vi "Dashboard Main.vi"() -> ()   [LabVIEW 2013]
uses:
  Robot Code/2014 Initial Robot/Shooter State Enum.ctl
  <vilib>/event_ctls.llb/eventvkey.ctl
  <vilib>/Rock Robotics/WPI/Dashboard/WPI_DashboardLogging Global.vi
  <vilib>/Utility/config.llb/Write Key (String).vi
  <vilib>/Utility/config.llb/Write Key (I32).vi
  <vilib>/Utility/config.llb/NI_LVConfig.lvlib
panel:
  out "Image Message":string="Timeout in Camera Communications"
  in  "Rec Mode":enum32{"Stop", "Record", "Playback"}(radio)
  in  "Dashboard Tab":T1(tab)
  in  "Camera Settings":T2={"Frame Rate"=30, "Compression"=30, "Size"=1} {"Frame Rate" scale=1.0..30.0; "Size" items=["640x480", "320x240", "160x120"]}
  out "MotorSliders R":cluster{"MotorSlide1":dbl, "MotorSlide2":dbl} {"MotorSlide2" scale=-1.0..1.0 scale format="%#_2e"; "MotorSlide1" scale=-1.0..1.0 scale format="%#_2e"}
  out "MotorChart R":cluster{"Numeric":dbl, "Numeric":dbl}(graph)
  out "MotorSliders L":T3 {"MotorSlide4 2" scale=0.0..14.0 scale format="%#_2e"; "MotorSlide2" scale=-1.0..1.0 scale format="%#_2e"; "MotorSlide1" scale=-1.0..1.0 scale format="%#_2e"}
  out "MotorChart L":T4(graph)
  out "JS1 Z":dbl(slide) scale=-1.0..1.0 scale format="%#_2e"
  out "Joystick 1":cluster{"X":dbl, "Y":dbl}[](graph)
  out "JS Buttons 1":T5
  out "JS2 Z":dbl(slide) scale=-1.0..1.0 scale format="%#_2e"
  out "Joystick 2":cluster{"X":dbl, "Y":dbl}[](graph)
  out "JS Buttons 2":T5
  out "Mode":T6(ring)=enum."Auto Disabled"
  out "Camera IP":string
  in  "DB Camera Config":bool
  out "fps":dbl format="%#.1g"
  out "Mbps":dbl format="%#.1g"
  out "Mbps 2":bool
  out "LED 1":bool
  out "Shooter":bool
  in  "ShotDrawSpeed":dbl format="%#_13g"
  in  "Pass Speed":dbl=1.0
  in  "Capture Speed":dbl=-1.0
  out "Pass":bool
  out "Collection Motors\nCapture":bool
  out "Upper":bool
  out "Limit Switches\nLower":bool
  in  "ArmSpeedDown":dbl=0.2
  in  "ArmSpeedUp":dbl=0.35
  out "ArmPosition":string
  out "CurrentPosition":dbl
  in  "TrussPosition":dbl=100.0
  in  "ShootPosition":dbl=61.0
  in  "PickUpPosition":dbl=12.0
  out "YAxisAccel":dbl
  in  "SecToFull":dbl=0.5 min=0.2 max=2.0
  out "ArmMotorValue":dbl
  out "Shooter State":T7
  in  "Checkbox 2":bool
  in  "Checkbox 1":bool
  in  "Test Slider":dbl(slide) scale=0.0..100.0 scale format="%#_3g"
  in  "On/Off":bool caption="Solenoid"
  in  "Test Name":u16(ring) items=["Select the test to run...", "Example Test", "-------------------------------", "List of tests is built in robot code.", "Replace with your own automated tests."]
  in  "Test Tree":string(tree)
  in  "Motor":cluster{"Value":dbl, "Enable":bool} {"Value" scale=-1.0..1.0 scale format="%#_3g"}
  out "Progress":T8 {"Test Progress" scale=0.0..100.0}
  in  "Rev/Fwd":cluster{"Forward":bool, "Reverse":bool}
  in  "Test Ring":u16(ring) items=["Auto", "Fixed indoor", "Fixed outdoor 1", "Fixed outdoor 2", "Fixed fluorescent 1", "Fixed fluorescent 2", "Hold current"]
  out "Potentiometer Value":dbl
  in  "Bottom Arm Value":dbl=1.43
  in  "Listbox":i32(listbox)
  out "Tree":string(tree)
  out "Camera Image":T9(plugin-control)
  in  "Enable":bool
  # "Left"
  # "Front"
  # "Right"
  # "Battery"
  # "This tab is a great place for autonomous settings and validation.\nCustomize by placing controls and indicators here and name to\nmatch Dashboard Variables on robot."
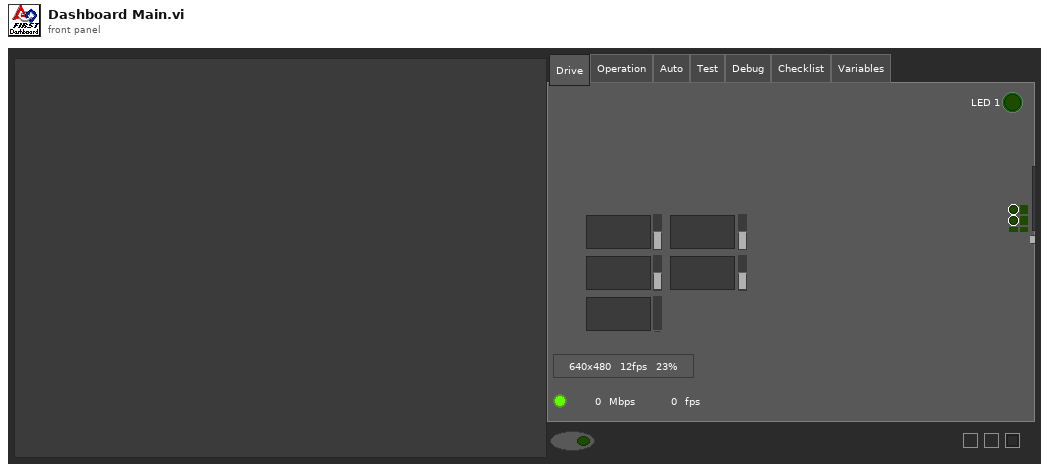
[diagram p1: front panel]
types:
  T1 = enum32{"Drive", "Operation", "Auto", "Test", "Debug", "Checklist", "Variables"}
  T2 = cluster{"Frame Rate":i32, "Compression":i32, "Size":u16}
  T3 = cluster{"MotorSlide1":dbl, "MotorSlide2":dbl, "MotorSlide4 2":dbl}
  T4 = cluster{"Numeric":dbl, "Numeric":dbl, "Battery":sgl}
  T5 = cluster{bool, bool, bool, bool, bool, bool, bool, bool, bool, bool, bool, bool}
  T6 = enum8{"Tele-Op Disabled", "Tele-Op Enabled", "Auto Disabled", "Auto Enabled", "Test Disabled", "Test Enabled", ""}
  T7 = typedef "Shooter State Enum.ctl" = enum16{"Ready", "Fired", "DrawingToReady"}
  T8 = cluster{"Test Progress":u8, "Test Progress Text":string}
  T9 = typedef "IMAQ Image.ctl" = refnum<image>
  T10 = enum32{"Drive", "Operation", "Auto", "Test", "Checklist", "Variables"}
  T11 = typedef "Image Type" = u32
  T12 = cluster{"Digital Inputs":bool[], "Digital Outputs":bool[]}
  T13 = cluster{"Competition mode":bool, "Robot Link":bool, "Autonomous":bool, "Enabled":bool, "E-Stop":bool, "Simulated":bool, "TestMode":bool, "Docked Window":bool}
  T14 = cluster{"Boolean Array[0]":bool, "Boolean Array[1]":bool, "Boolean Array[2]":bool, "Boolean Array[3]":bool, "Boolean Array[4]":bool, "Boolean Array[5]":bool, "Boolean Array[6]":bool, "Boolean Array[7]":bool, "Boolean Array[8]":bool, "Boolean Array[9]":bool, "Boolean Array[10]":bool, "Boolean Array[11]":bool}
  T15 = typedef "NI_LVConfig.lvlib/Config Data RefNum.ctl" = refnum<k1>
  T16 = typedef "eventvkey.ctl" = enum16{"ASCII", "Enter", "Return", "Shift", "Ctrl", "Alt", "Cmd", "Opt", "Caps", "NumLock", "Clear", "Break", "Up", "Down", "Left", "Right", "Insert", "Delete", "Home", "End", "PageUp", "PageDown", "Escape", "Help", "Pause", "ScrollLock", "F1", "F2", "F3", "F4", "F5", "F6", "F7", "F8", "F9", "F10", "F11", "F12", "F13", "F14", "F15", "F16", "F17", "F18", "F19", "F20", "F21", "F22", "F23", "F24", "Play", "VolumeUp", "VolumeDown", "Mute", "Two Byte Char"}
  T17 = cluster{"Image Size":bool, "Image Type":bool, "Pixel Value":bool, "ROI Information":bool, "Zoom Factor":bool}
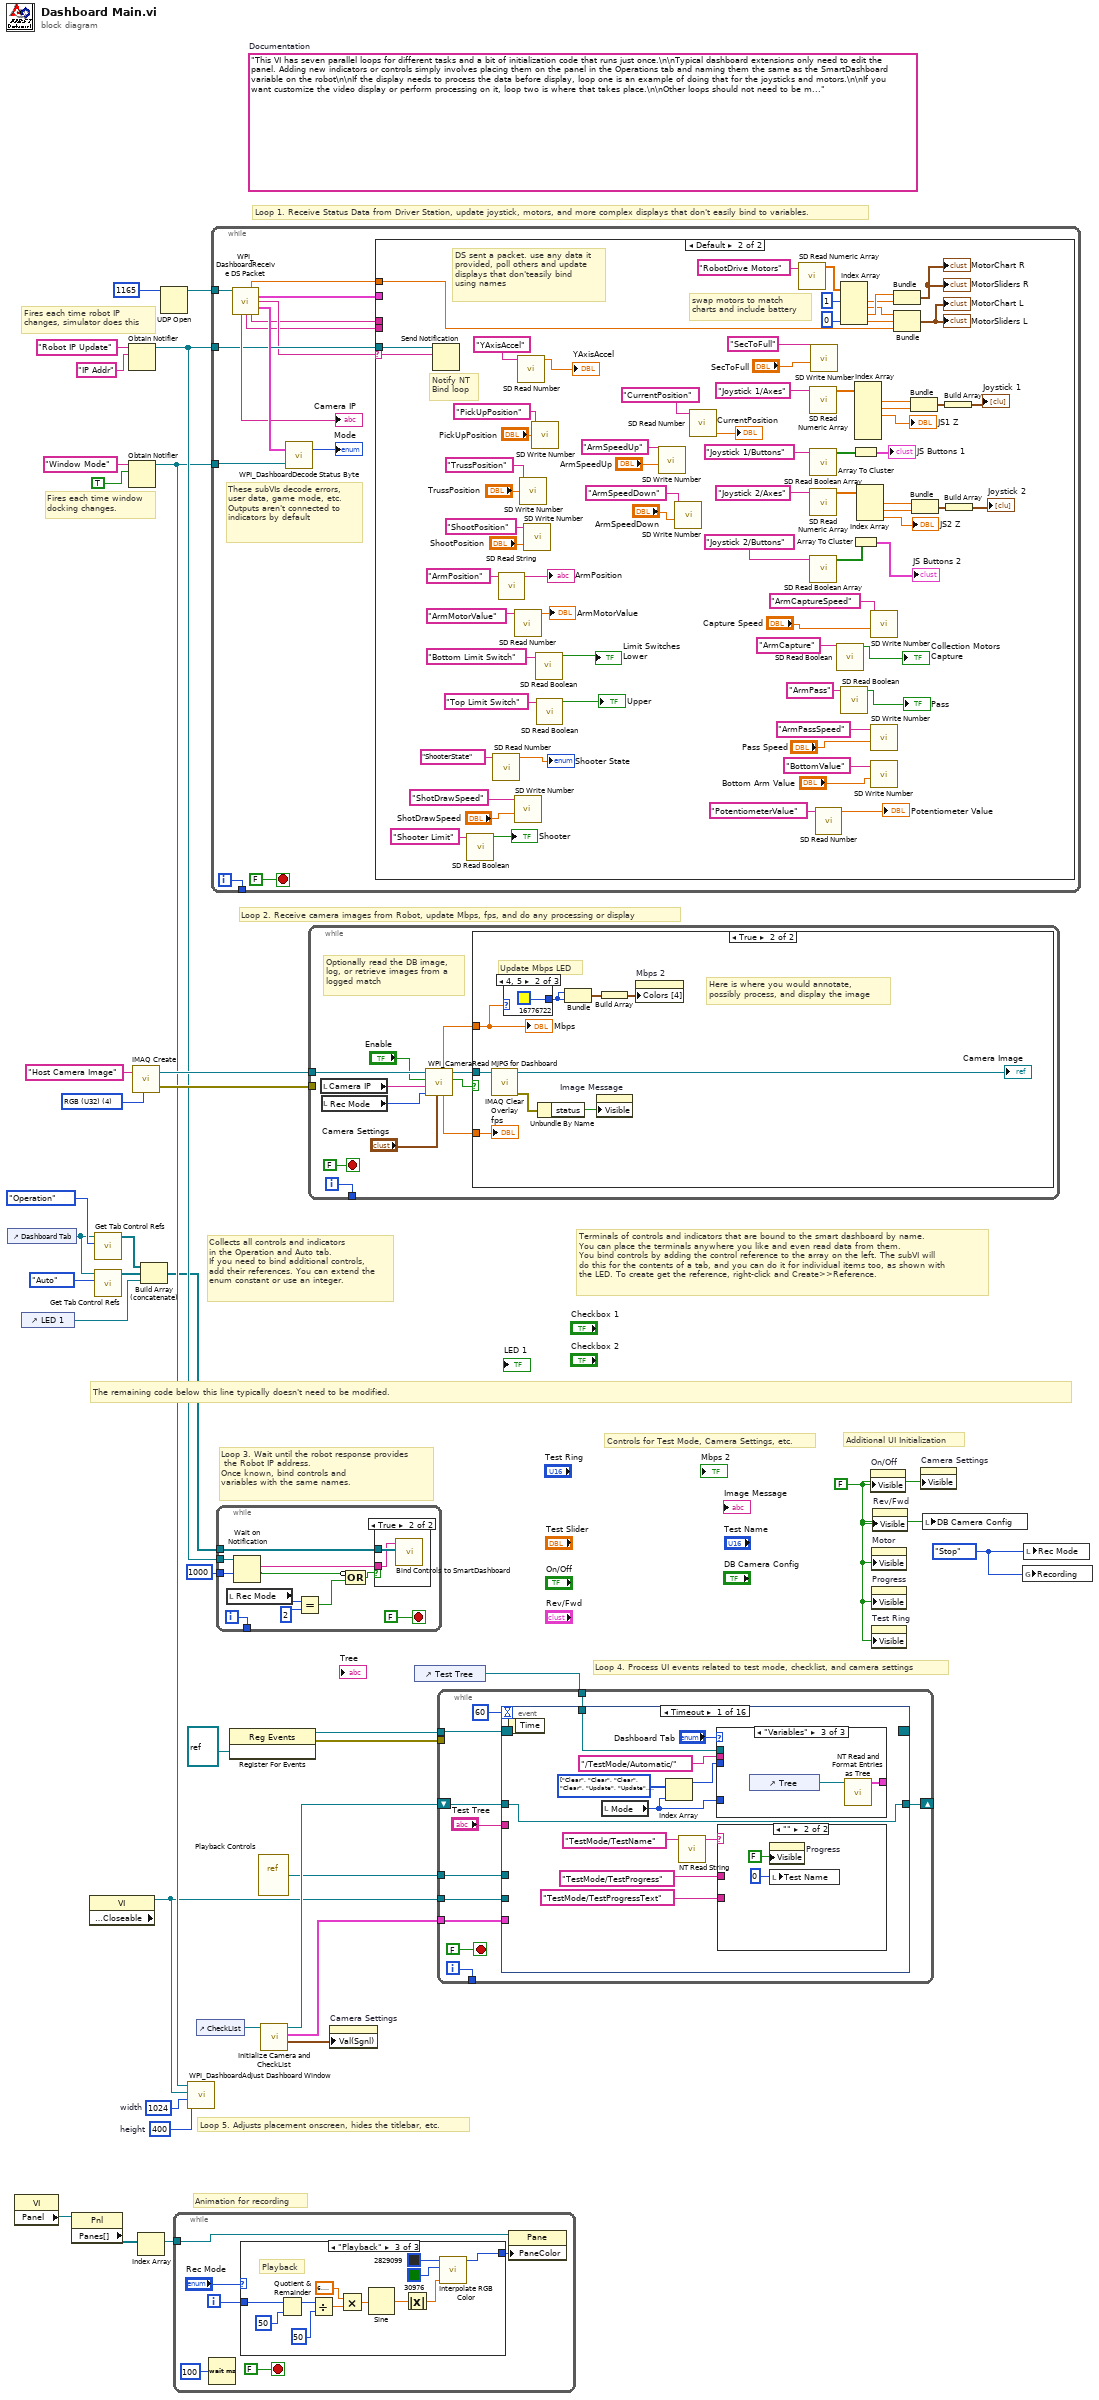
[diagram p0: block diagram]
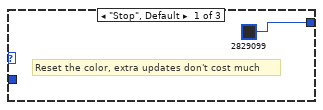
[diagram p2: hidden frame]
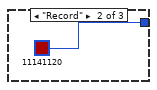
[diagram p3: hidden frame]
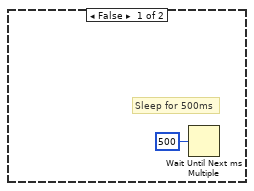
[diagram p5: hidden frame]
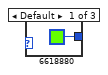
[diagram p6: hidden frame]
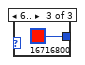
[diagram p7: hidden frame]
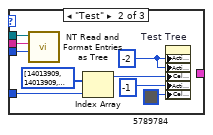
[diagram p9: hidden frame]
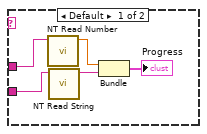
[diagram p10: hidden frame]
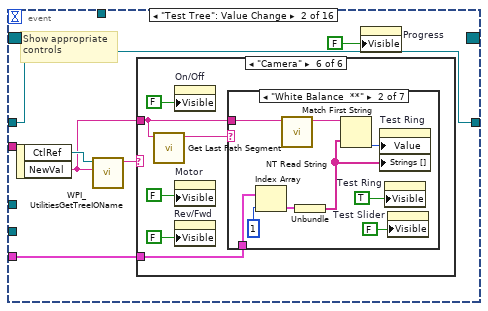
[diagram p11: hidden frame]
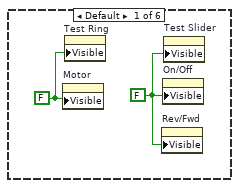
[diagram p12: hidden frame]
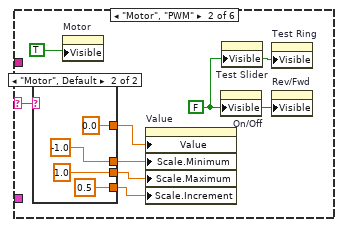
[diagram p13: hidden frame]
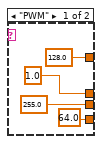
[diagram p14: hidden frame]
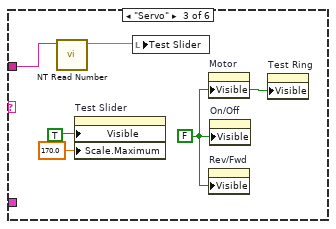
[diagram p15: hidden frame]
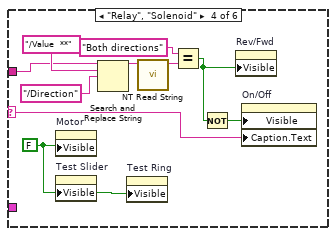
[diagram p16: hidden frame]
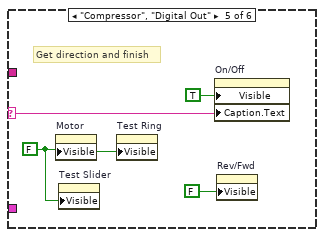
[diagram p17: hidden frame]
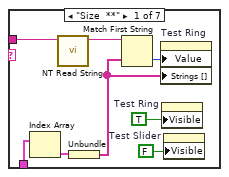
[diagram p18: hidden frame]
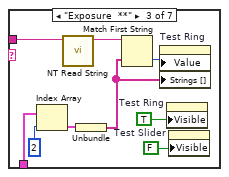
[diagram p19: hidden frame]
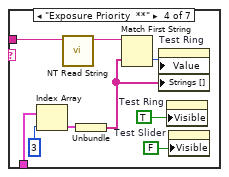
[diagram p20: hidden frame]
diagram:
  w8 = enum32{"Stop", "Record", "Playback"}."Stop" ("Rec Mode")
  w11 = 400  # height
  w12 = 1024  # width
  w25 = FALSE ("Visible")
  (unwired) "This VI has seven parallel loops for different tasks and a bit of initialization code that runs just once.\n\nTypical dashboard extensions only need to edit the panel. Adding new indicators or controls simply involves placing them on the panel in the Operations tab and naming them the same as the SmartDashboard variable on the robot\n\nIf the display needs to process the data before display, loop one is an example of doing that for the joysticks and motors.\n\nIf you want customize the video display or perform processing on it, loop two is where that takes place.\n\nOther loops should not need to be modified. They are pretty standard, and document the task they perform."  # Documentation
  w35 = T11 4 items=["Grayscale (U8)", "Grayscale (I16)", "Grayscale (SGL)", "Complex (CSG)", "RGB (U32)", "HSL (U32)", "RGB (U64)"] ("Image Type")
  # "Controls for Test Mode, Camera Settings, etc."
  # "Additional UI Initialization"
  # "Animation for recording"
  # "Fires each time robot IP\nchanges, simulator does this"
  # "Fires each time window\ndocking changes."
  # "Collects all controls and indicators\nin the Operation and Auto tab.\nIf you need to bind additional controls,\nadd their references. You can extend the\nenum constant or use an integer."
  # "The remaining code below this line typically doesn't need to be modified."
  # "Loop 4. Process UI events related to test mode, checklist, and camera settings"
  # "Terminals of controls and indicators that are bound to the smart dashboard by name.\nYou can place the terminals anywhere you like and even read data from them.\nYou bind controls by adding the control reference to the array on the left. The subVI will\ndo this for the contents of a tab, and you can do it for individual items too, as shown with\nthe LED. To create get the reference, right-click and Create>>Reference."
  # "Loop 3. Wait until the robot response provides\n the Robot IP address.\nOnce known, bind controls and\nvariables with the same names."
  # "Loop 5. Adjusts placement onscreen, hides the titlebar, etc."
  # "Loop 1. Receive Status Data from Driver Station, update joystick, motors, and more complex displays that don't easily bind to variables."
  # "Loop 2. Receive camera images from Robot, update Mbps, fps, and do any processing or display"
  n1 = control-ref of="Dashboard Tab"() -> (w6:refnum<vi>)
  n2 = property class="VI"() -> ("Panel"=w19:refnum<vi>)  [unwired: 2 in, 2 out]
  n3 = control-ref of="LED 1"() -> (w1:refnum<vi>)
  n4 = property class="Pnl"(reference=w19) -> ("Panes[]"=w20:refnum<vi>[])  [unwired: 1 in, 2 out]
  n5 = property class="VI" props=["Front Panel.Closeable"]() -> (reference out=w7:refnum<vi>)  [unwired: 2 in, 2 out]
  n6 = call <vilib>:"Get Tab Control Refs.vi"("Page Index"=T10."Operation" ("Dashboard Tab"), "TabControl in"=w6) -> ("ControlsOnPage"=w4:refnum<vi>[])  [unwired: 9 in]
  n7 = call <vilib>:"Get Tab Control Refs.vi"("Page Index"=T10."Auto" ("Dashboard Tab"), "TabControl in"=w6) -> ("ControlsOnPage"=w5:refnum<vi>[])  [unwired: 9 in]
  n8 = Obtain Notifier(name (unnamed)="Robot IP Update", notification data type="IP Addr" ("name (unnamed)")) -> (notifier out=w29:refnum<notifier>)  [unwired: 2 in, 2 out]
  n9 = Obtain Notifier(name (unnamed)="Window Mode", notification data type=TRUE) -> (notifier out=w10:refnum<notifier>)  [unwired: 2 in, 2 out]
  n10 = call "IMAQ Create"("Image Name"="Host Camera Image", "Image Type"=w35) -> ("New Image"=w33:T9, "error out"=w32:errorcluster)  [unwired: 2 in, 1 out]
  n11 = Index Array(array=w20) -> (element=w18:refnum<vi>)  [unwired: 1 in]
  n12 = Build Array (concatenate)(w4, w5, w1) -> (w3:refnum<vi>[])
  n13 = UDP Open(11:u16 1165 ("port")) -> (port=w36:refnum<k16>)  [unwired: 2 in, 4 out]
  n14 = while {
    tunnel: w18 -> [w39]
    i -> [w42]
    stop <- FALSE stop-if-true
    n15 = Wait (ms)(milliseconds to wait=u32 100) -> ()  [unwired: 1 out]
    n16 = case shown="\"Playback\"" "Rec Mode" {
      tunnel: w42 -> [_ _ w57]
      tunnel: [u32 2829099 ("Base Color") u32 11141120 ("Target Color") w46] -> w38
      frame "Stop", Default {
        # "Reset the color, extra updates don't cost much"
      }
      frame "Record" {
      }
      frame "Playback" {
        # "Playback"
        n17 = Quotient & Remainder(x=w57, y=u32 50 ("milliseconds to wait")) -> (x-y*floor(x/y)=w53:u32)  [unwired: 1 out]
        n18 = Divide(x=w53, y=u32 50 ("milliseconds to wait")) -> (x/y=w50:dbl)
        n19 = Multiply(x=6.283185307179586, y=w50) -> (x*y=w55:dbl)
        n20 = Sine(x=w55) -> (sin(x)=w54:dbl)
        n21 = Absolute Value(x=w54) -> (abs(x)=w47:dbl)
        n22 = call "Interpolate RGB Color.vi"("Proportion"=w47, "Target Color"=u32 30976, "Base Color"=u32 2829099) -> ("Result Color"=w46:u32)  [unwired: 8 in]
      }
    }
    n23 = property class="Pane"(reference=w39, "PaneColor"=w38) -> ()  [unwired: 1 in, 2 out]
  }
  n24 = call <vilib>:"WPI_DashboardAdjust Dashboard Window.vi"("height"=w11, "width"=w12, "reference in"=w7, "Notifier in"=w10) -> ()  [unwired: 8 in]
  n25 = control-ref of="CheckList"() -> (w9:refnum<vi>)
  n26 = while {
    tunnel: w36 -> [w68]
    tunnel: w29 -> [w63]
    tunnel: w10 -> [w67]
    tunnel: [w64] -> _
    i -> [w64]
    stop <- FALSE stop-if-true
    # "These subVIs decode errors, user data, game mode, etc.\nOutputs aren't connected to indicators by default"
    n27 = call <vilib>:"WPI_DashboardReceive DS Packet.vi"("Recv Socket"=w68) -> ("Battery"=w58:sgl, "Driver Station"=w59:T12, "Robot IP Address"=w62:string, "Status"=w69:T13, "Camera IP Address"=→"Camera IP":string, "Low Priority User Data"=w61:string, "High Priority User Data"=w60:string)  [unwired: 1 in, 7 out]
    n28 = call <vilib>:"WPI_DashboardDecode Status Byte.vi"("Window Mode Notifier"=w67, "Status"=w69) -> ("Mode"=→"Mode":T6)  [unwired: 1 out]
    n29 = case shown="Default" w62 {
      selector: w62 -> [_ w123]
      tunnel: w63 -> [_ w124]
      tunnel: w61 -> [_ _]
      tunnel: w60 -> [_ _]
      tunnel: w59 -> [_ _]
      tunnel: w58 -> [_ w122]
      frame "0.0.0.0" {
        # "DS not sending packets, or no robot exists yet.\nDon't poll the variables"
      }
      frame Default {
        # "Notify NT\nBind loop"
        # "DS sent a packet. use any data it\nprovided, poll others and update\ndisplays that don'teasily bind\nusing names"
        # "swap motors to match\ncharts and include battery"
        n30 = Send Notification(notification=w123, notifier=w124) -> ()  [unwired: 1 in, 2 out]
        n31 = call <vilib>:"SD Read Boolean.vi"("Name"="Shooter Limit") -> ("Boolean"=→"Shooter":bool)  [unwired: 8 in, 2 out]
        n32 = call <vilib>:"SD Read Number.vi"("Name"="ShooterState") -> ("Numeric"=→"Shooter State":dbl)  [unwired: 8 in, 2 out]
        n33 = call <vilib>:"SD Read String.vi"("Name"="ArmPosition") -> ("String"=→"ArmPosition":string)  [unwired: 8 in, 2 out]
        n34 = call <vilib>:"SD Read Number.vi"("Name"="ArmMotorValue") -> ("Numeric"=→"ArmMotorValue":dbl)  [unwired: 8 in, 2 out]
        n35 = call <vilib>:"SD Write Number.vi"("Numeric"="ShotDrawSpeed", "Name"="ShotDrawSpeed") -> ()  [unwired: 8 in, 2 out]
        n36 = call <vilib>:"SD Read Number.vi"("Name"="YAxisAccel") -> ("Numeric"=→"YAxisAccel":dbl)  [unwired: 8 in, 2 out]
        n37 = call <vilib>:"SD Write Number.vi"("Numeric"="TrussPosition", "Name"="TrussPosition") -> ()  [unwired: 8 in, 2 out]
        n38 = call <vilib>:"SD Write Number.vi"("Numeric"="ShootPosition", "Name"="ShootPosition") -> ()  [unwired: 8 in, 2 out]
        n39 = call <vilib>:"SD Write Number.vi"("Numeric"="PickUpPosition", "Name"="PickUpPosition") -> ()  [unwired: 8 in, 2 out]
        n40 = call <vilib>:"SD Read Boolean.vi"("Name"="Bottom Limit Switch") -> ("Boolean"=→"Limit Switches\nLower":bool)  [unwired: 8 in, 2 out]
        n41 = call <vilib>:"SD Read Boolean.vi"("Name"="Top Limit Switch") -> ("Boolean"=→"Upper":bool)  [unwired: 8 in, 2 out]
        n42 = call <vilib>:"SD Write Number.vi"("Numeric"="ArmSpeedUp", "Name"="ArmSpeedUp") -> ()  [unwired: 8 in, 2 out]
        n43 = call <vilib>:"SD Write Number.vi"("Numeric"="ArmSpeedDown", "Name"="ArmSpeedDown") -> ()  [unwired: 8 in, 2 out]
        n44 = call <vilib>:"SD Read Number.vi"("Name"="CurrentPosition") -> ("Numeric"=→"CurrentPosition":dbl)  [unwired: 8 in, 2 out]
        n45 = call <vilib>:"SD Read Numeric Array.vi"("Name"="RobotDrive Motors") -> ("Numeric Array"=w121:dbl[])  [unwired: 8 in, 2 out]
        n46 = call <vilib>:"SD Read Numeric Array.vi"("Name"="Joystick 1/Axes") -> ("Numeric Array"=w140:dbl[])  [unwired: 8 in, 2 out]
        n47 = call <vilib>:"SD Read Boolean Array.vi"("Name"="Joystick 1/Buttons") -> ("Boolean Array"=w142:bool[])  [unwired: 8 in, 2 out]
        n48 = call <vilib>:"SD Read Numeric Array.vi"("Name"="Joystick 2/Axes") -> ("Numeric Array"=w134:dbl[])  [unwired: 8 in, 2 out]
        n49 = call <vilib>:"SD Read Boolean Array.vi"("Name"="Joystick 2/Buttons") -> ("Boolean Array"=w133:bool[])  [unwired: 8 in, 2 out]
        n50 = call <vilib>:"SD Write Number.vi"("Numeric"="SecToFull", "Name"="SecToFull") -> ()  [unwired: 8 in, 2 out]
        n51 = call <vilib>:"SD Read Number.vi"("Name"="PotentiometerValue") -> ("Numeric"=→"Potentiometer Value":dbl)  [unwired: 8 in, 2 out]
        n52 = call <vilib>:"SD Read Boolean.vi"("Name"="ArmCapture") -> ("Boolean"=→"Collection Motors\nCapture":bool)  [unwired: 8 in, 2 out]
        n53 = Index Array(array=w121, index #1=1, index #4=0) -> (element #1=w117:dbl, element #2=w116:dbl, element #3=w118:dbl, element #4=w113:dbl)  [unwired: 2 in]
        n54 = call <vilib>:"SD Read Boolean.vi"("Name"="ArmPass") -> ("Boolean"=→"Pass":bool)  [unwired: 8 in, 2 out]
        n55 = Array To Cluster(array=w142) -> (cluster=→"JS Buttons 1":T14)
        n56 = Array To Cluster(array=w133) -> (cluster=→"JS Buttons 2":T14)
        n57 = Index Array(array=w140) -> (element #1=w137:dbl, element #2=w138:dbl, element #3=→"JS1 Z":dbl)  [unwired: 6 in, 3 out]
        n58 = Index Array(array=w134) -> (element #1=w129:dbl, element #2=w128:dbl, element #3=→"JS2 Z":dbl)  [unwired: 3 in]
        n59 = call <vilib>:"SD Write Number.vi"("Numeric"="Capture Speed", "Name"="ArmCaptureSpeed") -> ()  [unwired: 8 in, 2 out]
        n60 = call <vilib>:"SD Write Number.vi"("Numeric"="Pass Speed", "Name"="ArmPassSpeed") -> ()  [unwired: 8 in, 2 out]
        n61 = call <vilib>:"SD Write Number.vi"("Numeric"="Bottom Arm Value", "Name"="BottomValue") -> ()  [unwired: 8 in, 2 out]
        n62 = Bundle("Numeric"=w118, "Numeric"=w117) -> (→"MotorChart R" →"MotorSliders R":cluster{"Numeric":dbl, "Numeric":dbl})  [unwired: 1 in]
        n63 = Bundle("Numeric"=w116, "Numeric"=w113, "Battery"=w122) -> (→"MotorChart L" →"MotorSliders L":T4)  [unwired: 1 in]
        n64 = Bundle("Numeric"=w137, "Numeric"=w138) -> (w136:cluster{"Numeric":dbl, "Numeric":dbl})  [unwired: 1 in]
        n65 = Bundle("Numeric"=w129, "Numeric"=w128) -> (w130:cluster{"Numeric":dbl, "Numeric":dbl})  [unwired: 1 in]
        n66 = Build Array(w136) -> (→"Joystick 1":cluster{"Numeric":dbl, "Numeric":dbl}[])
        n67 = Build Array(w130) -> (→"Joystick 2":cluster{"Numeric":dbl, "Numeric":dbl}[])
      }
    }
  }
  n68 = while {
    tunnel: w3 -> [w156]
    tunnel: w29 -> [w154]
    tunnel: [w152] -> _
    tunnel: u32 1000 ("milliseconds to wait") -> [w151]
    i -> [w152]
    stop <- FALSE stop-if-true
    n69 = local read "Rec Mode"() -> (w147:enum32{"Stop", "Record", "Playback"})
    n70 = Wait on Notification(notifier=w154, timeout in ms (-1)=w151) -> (notification=w153:string, timed out?=w149:bool)  [unwired: 2 in, 2 out]
    n71 = Equal?(x=w147, y=u16 2 ("Rec Mode")) -> (x = y?=w148:bool)
    n72 = Compound Arithmetic op=OR(invert w149, w148) -> (w150:bool)
    n73 = case shown="True" w150 {
      tunnel: w156 -> [_ w158]
      tunnel: w153 -> [_ w157]
      frame False {
      }
      frame True {
        n74 = call <vilib>:"Bind Controls to SmartDashboard.vi"("Bound Control Refs"=w158, "Server IP Address"=w157) -> ()  [unwired: 10 in]
      }
    }
  }
  n75 = register-events(refnum<vi> refnum) -> (reference out=w16:refnum<event-registration>, error out=w15:errorcluster)  [unwired: 2 in]
  n76 = vi-ref "Playback Controls.vi"() -> (w17:refnum<vi>)
  n77 = call "Initialize Camera and CheckList.vi"("ListBox in"=w9) -> ("Cluster"=w23:cluster{"value":i32, "value":i32, "index":i32}, "Array"=w24:cluster{string[]}[], "File Refnum"=w22:T15)  [unwired: 8 in]
  n78 = while {
    tunnel: w33 -> [w167]
    tunnel: w32 -> [_]
    tunnel: [w168] -> _
    i -> [w168]
    stop <- FALSE stop-if-true
    # "Optionally read the DB image,\nlog, or retrieve images from a\nlogged match"
    n79 = local read "Camera IP"() -> (w160:string)
    n80 = local read "Rec Mode"() -> (w159:enum32{"Stop", "Record", "Playback"})
    n81 = call <vilib>:"WPI_CameraRead MJPG for Dashboard.vi"("Camera Settings"="Camera Settings", "Rec Mode"=w159, "Camera IP"=w160, "Enable"="Enable", "Refnum in"=w167) -> ("Active"=w164:bool, "Refnum out"=w166:T9, "FPS"=w163:dbl, "Bandwidth (Mbps)"=w162:dbl)  [unwired: 3 in]
    n82 = case shown="True" w164 {
      tunnel: w166 -> [_ w174]
      tunnel: w162 -> [_ w173]
      tunnel: w163 -> [_ w171]
      frame False {
        # "Sleep for 500ms"
        n83 = Wait Until Next ms Multiple(millisecond multiple=u32 500) -> ()  [unwired: 1 out]
      }
      frame True {
        # "Here is where you would annotate,\npossibly process, and display the image"
        # "Update Mbps LED"
        n84 = call "IMAQ Clear Overlay"("Image"=w174) -> ("error out"=w178:errorcluster, "Image Out"=→"Camera Image":T9)  [unwired: 2 in, 7 out]
        n85 = case shown="4, 5" w173 {
          tunnel: [u32 6618880 ("Color Box") u32 16776722 ("Color Box") u32 16716800 ("Color Box")] -> w175
          frame Default {
          }
          frame 4, 5 {
          }
          frame 6.. {
          }
        }
        n86 = Unbundle By Name(w178) -> ("status"=w179:bool)
        n87 = Bundle("Color Box"=w175, "Color Box"=w175) -> (w177:cluster{"Color Box":u32, "Color Box":u32})  [unwired: 1 out]
        n88 = property on="Image Message" class="Str"("Visible"=w179) -> ()  [unwired: 2 in, 2 out]
        n89 = Build Array(w177) -> (w176:cluster{"Color Box":u32, "Color Box":u32}[])
        n90 = property on="Mbps 2" class="Bool (strict)"("Colors [4]"=w176) -> ()  [unwired: 2 in, 2 out]
        "Mbps" <- w173
        "fps" <- w171
      }
    }
  }
  n91 = property on="Camera Settings" class="Clust (strict)"("Val(Sgnl)"=w23) -> ()  [unwired: 2 in, 2 out]
  n92 = control-ref of="Test Tree"() -> (w21:refnum<vi>)
  n93 = while {
    tunnel: w24 -> [w190]
    shift-right: [w189] -> _
    shift-left: w22 -> [w188]
    tunnel: [w187] -> _
    tunnel: w21 -> [w186]
    tunnel: w17 -> [w185]
    tunnel: w16 -> [w184]
    tunnel: w15 -> [_]
    tunnel: w7 -> [w183]
    i -> [w187]
    stop <- FALSE stop-if-true
    n94 = event shown="[0] Timeout" {
      selector: w184 -> [_ _ _ _ _ _ _ _ _ _ _ _ _ _ _ _]
      dyn-events: [_ _ _ _ _ _ _ _ _ _ _ _ _ w428 _ _] -> _
      timeout: u32 60 ("milliseconds to wait") -> [_ _ _ _ _ _ _ _ _ _ _ _ _ _ _ _]
      tunnel: w186 -> [w200 _ _ _ _ _ _ _ _ _ _ _ _ _ _ _]
      tunnel: "Test Tree" -> [_ _ _ _ _ _ _ _ w397 w405 w407 w411 w419 _ _ _]
      tunnel: w190 -> [_ w224 _ _ _ _ w361 w391 _ _ _ _ _ _ _ _]
      tunnel: [w194 w223 w322 w327 w335 w347 w360 w384 w396 w403 w406 w410 w418 w430 w444 w445] -> w189
      tunnel: w188 -> [w194 w223 w322 w327 w335 w347 w359 w384 w396 w403 w406 w410 w418 w430 w444 w445]
      tunnel: w185 -> [_ _ _ _ _ _ _ _ _ _ _ _ _ w431 _ w448]
      tunnel: w183 -> [_ _ _ _ _ _ _ _ _ _ _ _ _ w426 _ _]
      event Timeout {
        w199 = enum16{"Update", "Clear"}[] [enum."Clear", enum."Clear", enum."Clear", enum."Clear", enum."Update", enum."Update", enum."Clear"] items=["Update", "Clear"]
        n95 = event-data() -> ()  [unwired: 1 in, 1 out]
        n96 = local read "Mode"() -> (w197:T6)
        n97 = Index Array(array=w199, index=w197) -> (element=w198:enum16{"Update", "Clear"})
        n98 = call <vilib>:"NT Read String.vi"("Name"="TestMode/TestName") -> ("String"=w203:string)  [unwired: 9 in, 1 out]
        n99 = case shown="\"Variables\"" "Dashboard Tab" {
          tunnel: w200 -> [_ w213 _]
          tunnel: "/TestMode/Automatic/" ("Name Pattern") -> [_ w212 _]
          tunnel: w198 -> [_ w211 _]
          tunnel: w197 -> [_ w209 _]
          tunnel: [_ _ w215] -> _
          frame "Operation", Default {
          }
          frame "Test" {
            w208 = -2 ("Active Item:Row Number")
            n100 = call <vilib>:"NT Read and Format Entries as Tree.vi"("Operation"=w211, "Name Pattern"=w212, "Tree Refnum"=w213) -> ()  [unwired: 7 in, 2 out]
            n101 = Index Array(array=u32[] [14013909, 14013909, 14013909, 14013909, 14013909, 16777215, 14013909], index=w209) -> (element=w207:u32)
            n102 = property on="Test Tree" class="Tree (strict)"("Active Item Row Number"=w208, "ActiveColNum"=w208, "CellBG"=w207, "Active Item Row Number"=-1 ("Active Item:Row Number"), "CellBG"=u32 5789784 ("Color Box")) -> ()  [unwired: 2 in, 2 out]
          }
          frame "Variables" {
            n103 = control-ref of="Tree"() -> (w214:refnum<vi>)
            n104 = call <vilib>:"NT Read and Format Entries as Tree.vi"("Tree Refnum"=w214) -> ("Formatted Strings"=w215:cluster{"Name":string, "Value":string}[])  [unwired: 9 in, 1 out]
          }
        }
        n105 = case shown="\"\"" w203 {
          tunnel: "TestMode/TestProgress" ("Name") -> [w217 _]
          tunnel: "TestMode/TestProgressText" ("Name") -> [w216 _]
          frame Default {
            n106 = call <vilib>:"NT Read Number.vi"("Name"=w217) -> ("Numeric"=w218:dbl)  [unwired: 9 in, 1 out]
            n107 = call <vilib>:"NT Read String.vi"("Name"=w216) -> ("String"=w219:string)  [unwired: 9 in, 1 out]
            n108 = Bundle("Numeric"=w218, "String"=w219) -> (→"Progress":cluster{"Numeric":dbl, "String":string})  [unwired: 1 in]
          }
          frame "" {
            n109 = property on="Progress" class="Clust (strict)"("Visible"=FALSE) -> ()  [unwired: 2 in, 2 out]
            n110 = local write "Test Name"(u16 0) -> ()
          }
        }
      }
      event "Test Tree": Value Change {
        # "Show appropriate\ncontrols"
        n111 = event-data() -> ("CtlRef"=w227:refnum<vi>, "NewVal"=w225:string)  [unwired: 1 in]
        n112 = call <vilib>:"WPI_UtilitiesGetTreeIOName.vi"("NewVal"=w225, "TreeControl in"=w227) -> ("I/O Name"=w228:string)  [unwired: 9 in]
        n113 = case shown="\"Camera\"" w228 {
          selector: w228 -> [_ w235 _ w253 w262 _]
          tunnel: w225 -> [_ _ w250 w252 _ w269]
          tunnel: w224 -> [_ _ _ _ _ w268]
          frame Default {
            w230 = FALSE ("Visible")
            w229 = FALSE ("Visible")
            n114 = property on="Motor" class="Clust (strict)"("Visible"=w229) -> ()  [unwired: 2 in, 2 out]
            n115 = property on="Test Ring" class="Ring (strict)"("Visible"=w229) -> ()  [unwired: 2 in, 2 out]
            n116 = property on="Rev/Fwd" class="Clust (strict)"("Visible"=w230) -> ()  [unwired: 2 in, 2 out]
            n117 = property on="On/Off" class="Bool (strict)"("Visible"=w230) -> ()  [unwired: 2 in, 2 out]
            n118 = property on="Test Slider" class="Slide (strict)"("Visible"=w230) -> ()  [unwired: 2 in, 2 out]
          }
          frame "Motor", "PWM" {
            w236 = FALSE ("Visible")
            n119 = case shown="\"Motor\", Default" w235 {
              tunnel: [1.0 ("Value") -1.0 ("Value")] -> w234
              tunnel: [255.0 ("Value") 1.0 ("Value")] -> w233
              tunnel: [128.0 ("Value") 0.0 ("Value")] -> w232
              tunnel: [64.0 ("Value") 0.5 ("Value")] -> w231
              frame "PWM" {
              }
              frame "Motor", Default {
              }
            }
            n120 = property on="Motor" class="Clust (strict)"("Visible"=TRUE) -> ()  [unwired: 2 in, 2 out]
            n121 = property on="Value" class="Slide (strict)"("Value"=w232, "Scale.Minimum"=w234, "Scale.Maximum"=w233, "Scale.Increment"=w231) -> ()  [unwired: 2 in, 2 out]
            n122 = property on="On/Off" class="Bool (strict)"("Visible"=w236) -> ()  [unwired: 2 in, 2 out]
            n123 = property on="Test Slider" class="Slide (strict)"("Visible"=w236) -> ()  [unwired: 2 in, 2 out]
            n124 = property on="Test Ring" class="Ring (strict)"("Visible"=w236) -> ()  [unwired: 2 in, 2 out]
            n125 = property on="Rev/Fwd" class="Clust (strict)"("Visible"=w236) -> ()  [unwired: 2 in, 2 out]
          }
          frame "Servo" {
            w248 = FALSE ("Visible")
            n126 = call <vilib>:"NT Read Number.vi"("Name"=w250) -> ("Numeric"=w249:dbl)  [unwired: 9 in, 1 out]
            n127 = property on="Test Slider" class="Slide (strict)"("Visible"=TRUE, "Scale.Maximum"=170.0 ("Scale.Range:Maximum")) -> ()  [unwired: 2 in, 2 out]
            n128 = local write "Test Slider"(w249) -> ()
            n129 = property on="Motor" class="Clust (strict)"("Visible"=w248) -> ()  [unwired: 2 in, 2 out]
            n130 = property on="Rev/Fwd" class="Clust (strict)"("Visible"=w248) -> ()  [unwired: 2 in, 2 out]
            n131 = property on="On/Off" class="Bool (strict)"("Visible"=w248) -> ()  [unwired: 2 in, 2 out]
            n132 = property on="Test Ring" class="Ring (strict)"("Visible"=w248) -> ()  [unwired: 2 in, 2 out]
          }
          frame "Relay", "Solenoid" {
            w251 = FALSE ("Visible")
            n133 = property on="Motor" class="Clust (strict)"("Visible"=w251) -> ()  [unwired: 2 in, 2 out]
            n134 = property on="Test Slider" class="Slide (strict)"("Visible"=w251) -> ()  [unwired: 2 in, 2 out]
            n135 = Search and Replace String(input string=w252, search string="/Value  **", replace string="/Direction") -> (result string=w258:string)  [unwired: 5 in, 3 out]
            n136 = property on="Test Ring" class="Ring (strict)"("Visible"=w251) -> ()  [unwired: 2 in, 2 out]
            n137 = call <vilib>:"NT Read String.vi"("Name"=w258) -> ("String"=w256:string)  [unwired: 9 in, 1 out]
            n138 = Equal?(x="Both directions", y=w256) -> (x = y?=w254:bool)
            n139 = Not(x=w254) -> (.not. x?=w255:bool)
            n140 = property on="Rev/Fwd" class="Clust (strict)"("Visible"=w254) -> ()  [unwired: 2 in, 2 out]
            n141 = property on="On/Off" class="Bool (strict)"("Visible"=w255, "Caption.Text"=w253) -> ()  [unwired: 2 in, 2 out]
          }
          frame "Compressor", "Digital Out" {
            w261 = FALSE ("Visible")
            # "Get direction and finish"
            n142 = property on="Motor" class="Clust (strict)"("Visible"=w261) -> ()  [unwired: 2 in, 2 out]
            n143 = property on="Test Slider" class="Slide (strict)"("Visible"=w261) -> ()  [unwired: 2 in, 2 out]
            n144 = property on="Test Ring" class="Ring (strict)"("Visible"=w261) -> ()  [unwired: 2 in, 2 out]
            n145 = property on="On/Off" class="Bool (strict)"("Visible"=TRUE, "Caption.Text"=w262) -> ()  [unwired: 2 in, 2 out]
            n146 = property on="Rev/Fwd" class="Clust (strict)"("Visible"=FALSE) -> ()  [unwired: 2 in, 2 out]
          }
          frame "Camera" {
            n147 = call <vilib>:"Get Last Path Segment.vi"("String in"=w269) -> ("String out"=w270:string)  [unwired: 10 in]
            n148 = property on="On/Off" class="Bool (strict)"("Visible"=FALSE) -> ()  [unwired: 2 in, 2 out]
            n149 = property on="Motor" class="Clust (strict)"("Visible"=FALSE) -> ()  [unwired: 2 in, 2 out]
            n150 = property on="Rev/Fwd" class="Clust (strict)"("Visible"=FALSE) -> ()  [unwired: 2 in, 2 out]
            n151 = case shown="\"White Balance  **\"" w270 {
              tunnel: w269 -> [w276 w285 w294 w303 w312 _ w318]
              tunnel: w268 -> [w274 w282 w291 w300 w309 _ _]
              frame "Size  **" {
                n152 = Index Array(array=w274) -> (element=w273:cluster{string[]})  [unwired: 1 in]
                n153 = call <vilib>:"NT Read String.vi"("Name"=w276) -> ("String"=w275:string)  [unwired: 9 in, 1 out]
                n154 = Unbundle(w273) -> (w271:string[])
                n155 = Match First String(2:w271, 3:w275) -> (0:w272:i32)  [unwired: 1 out]
                n156 = property on="Test Ring" class="Ring (strict)"("Value"=w272, "Strings []"=w271) -> ()  [unwired: 2 in, 2 out]
                n157 = property on="Test Ring" class="Ring (strict)"("Visible"=TRUE) -> ()  [unwired: 2 in, 2 out]
                n158 = property on="Test Slider" class="Slide (strict)"("Visible"=FALSE) -> ()  [unwired: 2 in, 2 out]
              }
              frame "White Balance  **" {
                n159 = Index Array(array=w282, index=1) -> (element=w283:cluster{string[]})
                n160 = call <vilib>:"NT Read String.vi"("Name"=w285) -> ("String"=w284:string)  [unwired: 9 in, 1 out]
                n161 = Unbundle(w283) -> (w280:string[])
                n162 = Match First String(2:w280, 3:w284) -> (0:w279:i32)  [unwired: 1 out]
                n163 = property on="Test Ring" class="Ring (strict)"("Value"=w279, "Strings []"=w280) -> ()  [unwired: 2 in, 2 out]
                n164 = property on="Test Ring" class="Ring (strict)"("Visible"=TRUE) -> ()  [unwired: 2 in, 2 out]
                n165 = property on="Test Slider" class="Slide (strict)"("Visible"=FALSE) -> ()  [unwired: 2 in, 2 out]
              }
              frame "Exposure  **" {
                n166 = Index Array(array=w291, index=2) -> (element=w292:cluster{string[]})
                n167 = call <vilib>:"NT Read String.vi"("Name"=w294) -> ("String"=w293:string)  [unwired: 9 in, 1 out]
                n168 = Unbundle(w292) -> (w288:string[])
                n169 = Match First String(2:w288, 3:w293) -> (0:w289:i32)  [unwired: 1 out]
                n170 = property on="Test Ring" class="Ring (strict)"("Value"=w289, "Strings []"=w288) -> ()  [unwired: 2 in, 2 out]
                n171 = property on="Test Ring" class="Ring (strict)"("Visible"=TRUE) -> ()  [unwired: 2 in, 2 out]
                n172 = property on="Test Slider" class="Slide (strict)"("Visible"=FALSE) -> ()  [unwired: 2 in, 2 out]
              }
              frame "Exposure Priority  **" {
                n173 = Index Array(array=w300, index=3) -> (element=w301:cluster{string[]})
                n174 = call <vilib>:"NT Read String.vi"("Name"=w303) -> ("String"=w302:string)  [unwired: 9 in, 1 out]
                n175 = Unbundle(w301) -> (w297:string[])
                n176 = Match First String(2:w297, 3:w302) -> (0:w298:i32)  [unwired: 1 out]
                n177 = property on="Test Ring" class="Ring (strict)"("Value"=w298, "Strings []"=w297) -> ()  [unwired: 2 in, 2 out]
                n178 = property on="Test Ring" class="Ring (strict)"("Visible"=TRUE) -> ()  [unwired: 2 in, 2 out]
                n179 = property on="Test Slider" class="Slide (strict)"("Visible"=FALSE) -> ()  [unwired: 2 in, 2 out]
              }
              frame "Color Enable  **" {
                n180 = Index Array(array=w309, index=4) -> (element=w310:cluster{string[]})
                n181 = call <vilib>:"NT Read String.vi"("Name"=w312) -> ("String"=w311:string)  [unwired: 9 in, 1 out]
                n182 = Unbundle(w310) -> (w306:string[])
                n183 = Match First String(2:w306, 3:w311) -> (0:w307:i32)  [unwired: 1 out]
                n184 = property on="Test Ring" class="Ring (strict)"("Value"=w307, "Strings []"=w306) -> ()  [unwired: 2 in, 2 out]
                n185 = property on="Test Ring" class="Ring (strict)"("Visible"=TRUE) -> ()  [unwired: 2 in, 2 out]
                n186 = property on="Test Slider" class="Slide (strict)"("Visible"=FALSE) -> ()  [unwired: 2 in, 2 out]
              }
              frame Default {
                n187 = property on="Test Ring" class="Ring (strict)"("Visible"=FALSE) -> ()  [unwired: 2 in, 2 out]
                n188 = property on="Test Slider" class="Slide (strict)"("Visible"=FALSE) -> ()  [unwired: 2 in, 2 out]
              }
              frame "Brightness  **", "Color Level  **", "Compression  **", "FPS  **", "Sharpness  **" {
                n189 = call <vilib>:"NT Read Number.vi"("Name"=w318) -> ("Numeric"=w317:dbl)  [unwired: 9 in, 1 out]
                n190 = local write "Test Slider"(w317) -> ()
                n191 = property on="Test Slider" class="Slide (strict)"("Visible"=TRUE, "Scale.Maximum"=100.0 ("Scale.Range:Maximum")) -> ()  [unwired: 2 in, 2 out]
                n192 = property on="Test Ring" class="Ring (strict)"("Visible"=FALSE) -> ()  [unwired: 2 in, 2 out]
              }
            }
          }
        }
        n193 = property on="Progress" class="Clust (strict)"("Visible"=FALSE) -> ()  [unwired: 2 in, 2 out]
      }
      event "Test Name": Mouse Enter {
        # "Populate the ring with the list of tests"
        n194 = event-data() -> ()  [unwired: 1 in, 1 out]
        n195 = call <vilib>:"NT Read String Array.vi"("Name"="TestMode/TestList") -> ("String Array"=w326:string[])  [unwired: 9 in, 1 out]
        n196 = Build Array (concatenate)("Select the test to run...", w326) -> (w325:string[])
        n197 = property on="Test Name" class="Ring (strict)"("Strings []"=w325) -> ()  [unwired: 2 in, 2 out]
      }
      event "Test Name": Value Change {
        w328 = FALSE ("Visible")
        # "Tell the robot the test name to run"
        n198 = event-data() -> ("NewVal"=w332:u16)  [unwired: 1 in]
        n199 = property on="Test Name" class="Ring (strict)"() -> ("Strings []"=w333:string[])  [unwired: 2 in, 2 out]
        n200 = local write "Progress"(T8 {"Test Progress"=0, "Test Progress Text"=""} ("Progress")) -> ()
        n201 = Index Array(array=w333, index=w332) -> (element=w331:string)
        n202 = call <vilib>:"NT Write String.vi"("String"=w331, "Name"="TestMode/TestName") -> ()  [unwired: 9 in, 1 out]
        n203 = property on="Progress" class="Clust (strict)"("Visible"=TRUE) -> ()  [unwired: 2 in, 2 out]
        n204 = property on="Motor" class="Clust (strict)"("Visible"=w328) -> ()  [unwired: 2 in, 2 out]
        n205 = property on="Test Slider" class="Slide (strict)"("Visible"=w328) -> ()  [unwired: 2 in, 2 out]
        n206 = property on="On/Off" class="Bool (strict)"("Visible"=w328) -> ()  [unwired: 2 in, 2 out]
        n207 = property on="Rev/Fwd" class="Clust (strict)"("Visible"=w328) -> ()  [unwired: 2 in, 2 out]
        n208 = property on="Test Ring" class="Ring (strict)"("Visible"=w328) -> ()  [unwired: 2 in, 2 out]
      }
      event "Listbox": Double Click {
        n209 = event-data() -> ("PlatMods.Shift"=w336:bool, "Row"=w338:i32)  [unwired: 1 in]
        n210 = case shown="True" w336 {
          tunnel: w338 -> [w342 _]
          tunnel: 1 -> [w341 _]
          frame False {
            n211 = property on="Listbox" class="LstBox (strict)"() -> ("Item Symbols"=w340:i32[])  [unwired: 2 in, 2 out]
            n212 = Replace Array Subset(array=w340, new element=w341, index=w342) -> (w339:i32[])
            n213 = property on="Listbox" class="LstBox (strict)"("Item Symbols"=w339) -> ()  [unwired: 2 in, 2 out]
          }
          frame True {
            w343 = 0 ("Top Row")
            n214 = property on="Listbox" class="LstBox (strict)"() -> ("Number of Rows"=w345:u32)  [unwired: 2 in, 2 out]
            n215 = Initialize Array(0, w345) -> (w344:i32[])
            n216 = property on="Listbox" class="LstBox (strict)"("Top Row"=w343, "Value"=w343, "Item Symbols"=w344) -> ()  [unwired: 2 in, 2 out]
          }
        }
      }
      event "Listbox": Key Down {
        n217 = event-data() -> ("VKey"=w349:T16)  [unwired: 1 in]
        n218 = case shown="\"Left\", \"Right\"" w349 {
          selector: w349 -> [w354 _]
          tunnel: eventvkey."Left" ("VKey") -> [w352 _]
          frame "Left", "Right" {
            n219 = Equal?(x=w352, y=w354) -> (x = y?=w353:bool)
            n220 = Select(t=0, s=w353, f=1) -> (s? t:f=w355:i32)
            n221 = property on="Listbox" class="LstBox (strict)"() -> ("Item Symbols"=w358:i32[])  [unwired: 2 in, 2 out]
            n222 = Replace Array Subset(array=w358, new element=w355, index="Listbox") -> (w357:i32[])
            n223 = property on="Listbox" class="LstBox (strict)"("Item Symbols"=w357) -> ()  [unwired: 2 in, 2 out]
          }
          frame Default {
          }
        }
      }
      event "DB Camera Config": Value Change {
        n224 = event-data() -> ("NewVal"=w362:bool)  [unwired: 1 in]
        n225 = case shown="False" w362 {
          tunnel: w361 -> [w371 _]
          tunnel: [w364 w382] -> w360
          tunnel: w359 -> [w363 w382]
          frame False {
            w378 = "Camera"
            w381 = FALSE ("Visible")
            n226 = local read "Camera Settings"() -> (w370:T2)
            n227 = Index Array(array=w371) -> (element=w374:cluster{string[]})  [unwired: 1 in]
            n228 = Unbundle(w370) -> ("Frame Rate"=w369:i32, "Compression"=w368:i32, "Size"=w372:u16)
            n229 = Unbundle(w374) -> (w373:string[])
            n230 = Index Array(array=w373, index=w372) -> (element=w367:string)
            n231 = call-poly <vilib>:"Write Key.vi"("section"=w378, "value"=w367, "key"="Size", "refnum"=w363) -> ("refnum out"=w380:T15)  [unwired: 2 in, 5 out]
            n232 = call-poly <vilib>:"Write Key.vi"("section"=w378, "value"=w369, "key"="FrameRate", "refnum"=w380) -> ("refnum out"=w379:T15)  [unwired: 1 in, 6 out]
            n233 = property on="Camera Settings" class="Clust (strict)"("Visible"=w381) -> ()  [unwired: 2 in, 2 out]
            n234 = local write "DB Camera Config"(w381) -> ()
            n235 = call-poly <vilib>:"Write Key.vi"("section"=w378, "value"=w368, "key"="Compression", "refnum"=w379) -> ("refnum out"=w365:T15)  [unwired: 1 in, 6 out]
            n236 = call <vilib>:"Close Config Data.vi"("refnum"=w365) -> ("file path"=w366:path)  [unwired: 2 in, 8 out]
            n237 = call <vilib>:"Open Config Data.vi"("configuration file path"=w366) -> ("refnum"=w364:T15)  [unwired: 8 in, 2 out]
          }
          frame True {
            n238 = property on="Camera Settings" class="Clust (strict)"("Visible"=TRUE) -> ()  [unwired: 2 in, 2 out]
          }
        }
      }
      event "Camera Settings": Value Change {
        n239 = event-data() -> ("NewVal"=w395:T2)  [unwired: 1 in]
        n240 = Index Array(array=w391) -> (element=w390:cluster{string[]})  [unwired: 1 in]
        n241 = Unbundle(w395) -> ("Frame Rate"=w386:i32, "Compression"=w385:i32, "Size"=w388:u16)
        n242 = Unbundle(w390) -> (w389:string[])
        n243 = Index Array(array=w389, index=w388) -> (element=w387:string)
        n244 = Format Into String(format string="%s   %dfps   %d%%", w387, w386, w385) -> (resulting string=w392:string)  [unwired: 2 in, 1 out]
        n245 = Build Array(w392) -> (w393:string[])
        n246 = property on="DB Camera Config" class="Bool (strict)"("Strings [4]"=w393) -> ()  [unwired: 2 in, 2 out]
      }
      event "Motor.Enable": Value Change {
        n247 = event-data() -> ("NewVal"=w401:bool)  [unwired: 1 in]
        n248 = Unbundle("Motor") -> ("Value"=w400:dbl)  [unwired: 1 out]
        n249 = Select(t=w400, s=w401, f=0.0) -> (s? t:f=w398:dbl)
        n250 = call <vilib>:"NT Write Number.vi"("Numeric"=w398, "Name"=w397) -> ()  [unwired: 9 in, 1 out]
      }
      event "Test Slider": Value Change {
        n251 = event-data() -> ("NewVal"=w404:dbl)  [unwired: 1 in]
        n252 = call <vilib>:"NT Write Number.vi"("Numeric"=w404, "Name"=w405) -> ()  [unwired: 9 in, 1 out]
      }
      event "On/Off": Value Change {
        n253 = event-data() -> ("NewVal"=w409:bool)  [unwired: 1 in]
        n254 = Boolean To (0,1)(Boolean=w409) -> (0, 1=w408:i16)
        n255 = call <vilib>:"NT Write Number.vi"("Numeric"=w408, "Name"=w407) -> ()  [unwired: 9 in, 1 out]
      }
      event "Rev/Fwd": Value Change {
        n256 = event-data() -> ("NewVal.Forward"=w417:bool, "NewVal.Reverse"=w416:bool)  [unwired: 1 in]
        n257 = Boolean To (0,1)(Boolean=w417) -> (0, 1=w413:i16)
        n258 = Boolean To (0,1)(Boolean=w416) -> (0, 1=w415:i16)
        n259 = Negate(x=w415) -> (-x=w414:i16)
        n260 = Add(x=w413, y=w414) -> (x+y=w412:i16)
        n261 = call <vilib>:"NT Write Number.vi"("Numeric"=w412, "Name"=w411) -> ()  [unwired: 9 in, 1 out]
      }
      event "Test Ring": Value Change {
        n262 = event-data() -> ("NewVal"=w421:u16)  [unwired: 1 in]
        n263 = property on="Test Ring" class="Ring (strict)"() -> ("Strings []"=w422:string[])  [unwired: 2 in, 2 out]
        n264 = Index Array(array=w422, index=w421) -> (element=w420:string)
        n265 = call <vilib>:"NT Write String.vi"("String"=w420, "Name"=w419) -> ()  [unwired: 9 in, 1 out]
      }
      event "Rec Mode": Value Change {
        # "Update globals for recording mode and path to read log from.\nClear when logging and let NetworkTables set path for vision to\nuse."
        n266 = event-data() -> ("NewVal"=w432:enum32{"Stop", "Record", "Playback"})  [unwired: 1 in]
        n267 = global write "WPI_DashboardLogging Global.vi" "Logging Filename"(path "") -> ()
        n268 = case shown="\"Stop\", \"Record\"" w432 {
          tunnel: w431 -> [_ w434 w442]
          tunnel: [_ _ w441] -> w428
          tunnel: [_ _ w440] -> _
          tunnel: w426 -> [_ _ w438]
          tunnel: cluster{i32, i32} {-250, 170} -> [_ _ w437]
          tunnel: [_ _ T17 {"Image Size"=TRUE, "Image Type"=TRUE, "Pixel Value"=TRUE, "ROI Information"=TRUE, "Zoom Factor"=FALSE} ("Image Information Shown:All Elements")] -> w424
          tunnel: [_ _ TRUE ("Zoom Factor")] -> w423
          frame Default {
          }
          frame "Stop", "Record" {
            # "Place Window too"
            n269 = invoke class="VI" method="FP.Close"(reference=w434) -> (reference out=w433:refnum<vi>)  [unwired: 2 in, 2 out]
            n270 = invoke class="VI" method="Abort VI"(reference=w433) -> ()  [unwired: 2 in, 3 out]
          }
          frame "Playback" {
            n271 = call "Open Playback Panel.vi"("Offset"=w437, "DB VI Ref"=w438, "Playback in"=w442) -> ("Playback out"=w439:refnum<vi>)  [unwired: 8 in]
            n272 = register-events(w439) -> (reference out=w441:refnum<event-registration>, error out=w440:errorcluster)  [unwired: 2 in]
          }
        }
        n273 = global write "WPI_DashboardLogging Global.vi" "Recording"(w432) -> ()
        n274 = property on="Camera Image" class="ImageControl"("Image Information Shown"=w424, "Image Information Visible"=w423) -> ()  [unwired: 2 in, 2 out]
        n275 = call <vilib>:"WPI_DashboardNT Log FieldName Cache.vi"("Operation"=enum16{"Lookup/Add", "Index", "Clear"}."Clear") -> ()  [unwired: 8 in, 3 out]
      }
      event Panel Close {
        w443 = enum32{"Stop", "Record", "Playback"}."Stop" ("Rec Mode")
        n276 = event-data() -> ()  [unwired: 1 in, 4 out]
        n277 = local write "Rec Mode"(w443) -> ()
        n278 = global write "WPI_DashboardLogging Global.vi" "Recording"(w443) -> ()
      }
      event Panel Close {
        # "Abort playback window and ourself"
        n279 = event-data() -> ()  [unwired: 1 in, 4 out]
        n280 = invoke class="VI" method="FP.Close"(reference=w448) -> (reference out=w447:refnum<vi>)  [unwired: 2 in, 2 out]
        n281 = invoke class="VI" method="Abort VI"(reference=w447) -> (error out=w446:errorcluster)  [unwired: 2 in, 2 out]
        n282 = invoke class="VI" method="Abort VI"(error in=w446) -> ()  [unwired: 2 in, 3 out]
      }
    }
  }
  n283 = property on="On/Off" class="Bool (strict)"("Visible"=w25) -> ()  [unwired: 2 in, 2 out]
  n284 = property on="Motor" class="Clust (strict)"("Visible"=w25) -> ()  [unwired: 2 in, 2 out]
  n285 = property on="Progress" class="Clust (strict)"("Visible"=w25) -> ()  [unwired: 2 in, 2 out]
  n286 = property on="Test Ring" class="Ring (strict)"("Visible"=w25) -> ()  [unwired: 2 in, 2 out]
  n287 = property on="Rev/Fwd" class="Clust (strict)"("Visible"=w25) -> ()  [unwired: 2 in, 2 out]
  n288 = property on="Camera Settings" class="Clust (strict)"("Visible"=w25) -> ()  [unwired: 2 in, 2 out]
  n289 = local write "DB Camera Config"(w25) -> ()
  n290 = global write "WPI_DashboardLogging Global.vi" "Recording"(w8) -> ()
  n291 = local write "Rec Mode"(w8) -> ()
